vi "String Array to UDcluster Array.vi"(8 "error in (no error)":errorcluster, 11 "Array 3":string[](array[string])) -> (0 "error out":errorcluster, 3 "Array":T1[](array[typedef]))   [LabVIEW 2012]
uses:
  typedef/User_Data_Cluster.ctl
  typedef/User Accounts.ctl
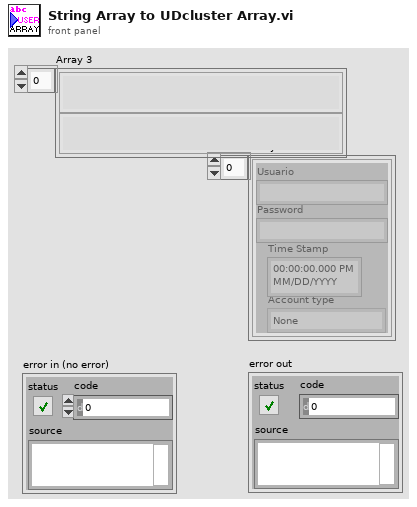
[diagram p1: front panel]
types:
  T1 = typedef "User_Data_Cluster.ctl" = cluster{"Usuario":string, "Password":string, "Account type":T2, "Time Stamp":timestamp}
  T2 = typedef "User Accounts.ctl" = enum16{"None", "User", "Admin"}
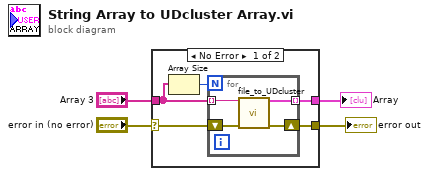
[diagram p0: block diagram]
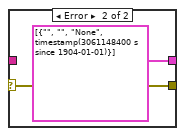
[diagram p2: hidden frame]
diagram:
  n1 = case shown="No Error" "error in (no error)" {
    selector: "error in (no error)" -> [w6 w14]
    tunnel: "Array 3" -> [w7 _]
    tunnel: [w9 T1[] [{"Usuario"="", "Password"="", "Account type"=enum."None", "Time Stamp"=timestamp(3061148400 s since 1904-01-01)}]] -> w2
    tunnel: [w5 w14] -> w4
    frame No Error {
      n2 = Array Size(array=w7) -> (size(s)=w8:i32)
      n3 = for {
        N: w8 -> [_]
        tunnel: [w13] -> w9 mode=indexing
        tunnel: w7 -> [w12] mode=indexing
        shift-right: [w11] -> w5
        shift-left: w6 -> [w10]
        n4 = call "file_to_UDcluster.vi"("Cyphered text"=w12, "error in (no error)"=w10) -> ("User-data cluster"=w13:T1, "error out"=w11:errorcluster)  [unwired: 12 in]
      }
    }
    frame Error {
    }
  }
  "error out" <- w4
  "Array" <- w2
